vi "State_Queue_Driver.vi"(0 "Queue_Name_In":string, 1 "Max_Queue_Size_In":i32=-1, 5 "State_In":string, 7 "N_State_In":string[](array[string]), 9 "Time_Out_In_ms (10)":i32=10, 11 "Error_In":errorcluster, 13 "Queue_Operation":T1=enum."Flush") -> (3 "Max_Queue_Size_Out":i32=-1, 4 "Queue_Name_Out":string, 6 "State_Out":string, 15 "Error_Out":errorcluster)   [LabVIEW 2021]
doc: "Used to transfer data from one state to another."
uses:
  Controls/Queue_Driver_Select.ctl
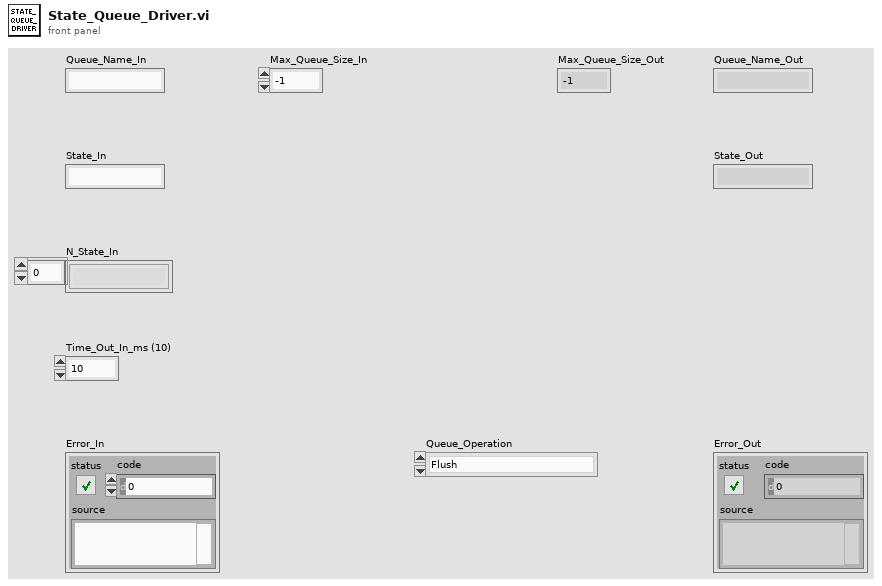
[diagram p1: front panel]
types:
  T1 = typedef "Queue_Driver_Select.ctl" = enum16{"Obtain_Queue", "Enqueue", "Enqueue_N", "Enqueue_at_Opposite_End", "Preview", "Queue_Status", "Dequeue", "Flush", "Release_Queue"}
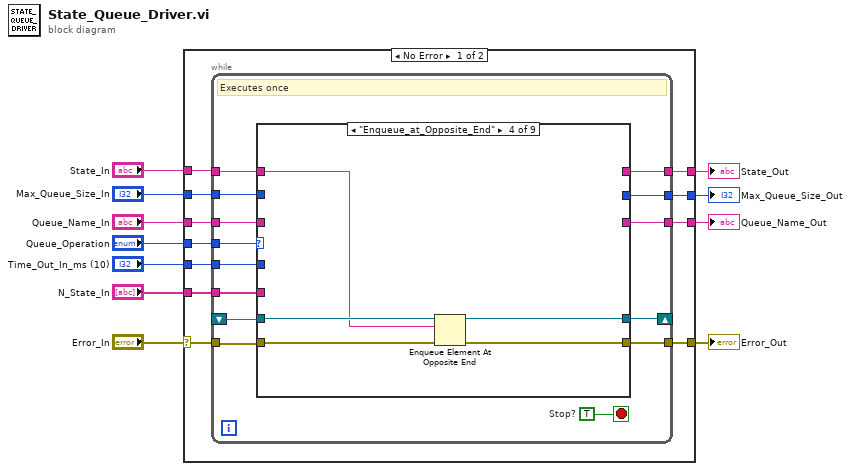
[diagram p0: block diagram]
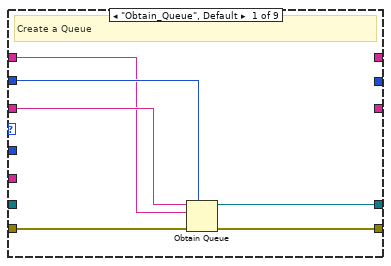
[diagram p2: hidden frame]
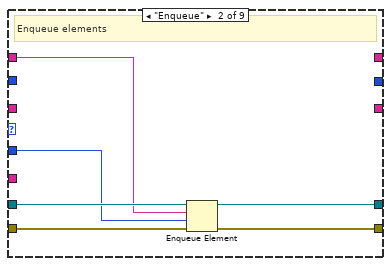
[diagram p3: hidden frame]
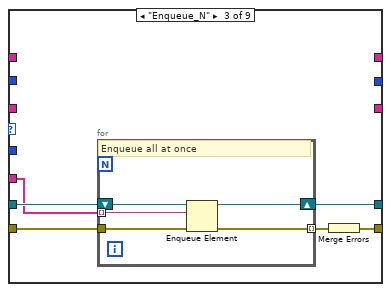
[diagram p4: hidden frame]
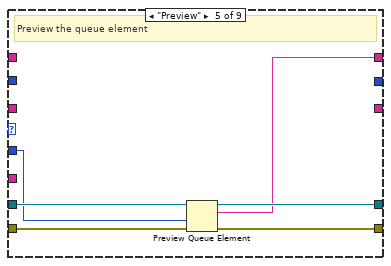
[diagram p5: hidden frame]
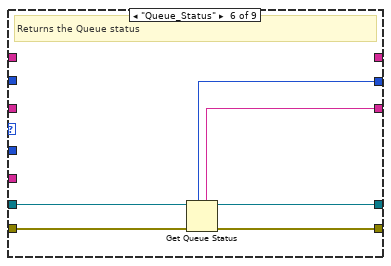
[diagram p6: hidden frame]
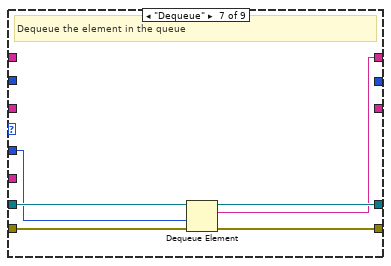
[diagram p7: hidden frame]
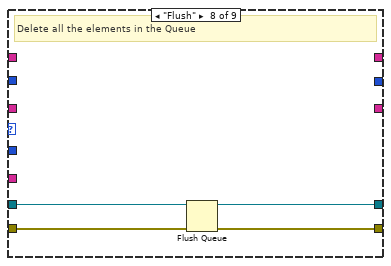
[diagram p8: hidden frame]
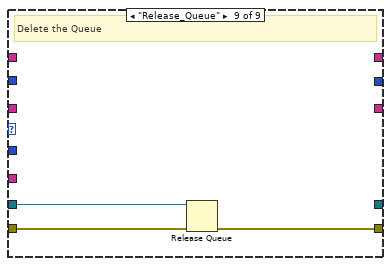
[diagram p9: hidden frame]
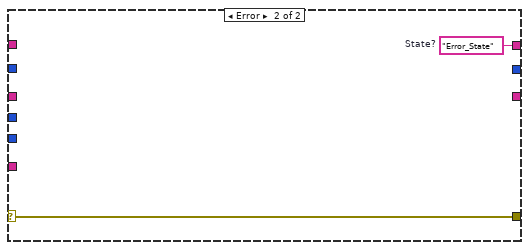
[diagram p10: hidden frame]
diagram:
  n1 = case shown="No Error" "Error_In" {
    selector: "Error_In" -> [w12 w91]
    tunnel: "Max_Queue_Size_In" -> [w22 _]
    tunnel: [w21 w91] -> w10
    tunnel: "Time_Out_In_ms (10)" -> [w20 _]
    tunnel: [w19 _] -> w8
    tunnel: [w18 _] -> w7
    tunnel: "Queue_Operation" -> [w17 _]
    tunnel: "Queue_Name_In" -> [w16 _]
    tunnel: "State_In" -> [w15 _]
    tunnel: [w14 w90] -> w3
    tunnel: "N_State_In" -> [w13 _]
    frame No Error {
      n2 = while {
        tunnel: w22 -> [w36]
        tunnel: w20 -> [w33]
        tunnel: [w31] -> w19
        tunnel: w17 -> [w28]
        shift-right: [w29] -> _
        shift-left: _ -> [w25]
        tunnel: w12 -> [w26]
        tunnel: [w35] -> w21
        tunnel: w13 -> [w23]
        tunnel: w15 -> [w34]
        tunnel: [w32] -> w14
        tunnel: w16 -> [w27]
        tunnel: [w30] -> w18
        stop <- w24 stop-if-true
        w24 = TRUE  # Stop?
        # "Executes once"
        n3 = case shown="\"Enqueue_at_Opposite_End\"" w28 {
          tunnel: w26 -> [w42 w48 w50 w63 w69 w75 w81 w85 w88]
          tunnel: w27 -> [w40 _ _ _ _ _ _ _ _]
          tunnel: w36 -> [w39 _ _ _ _ _ _ _ _]
          tunnel: [w37 w44 w53 w62 w68 w74 w80 w84 _] -> w29
          tunnel: [w41 w47 w49 w61 w67 w73 w78 w83 w87] -> w35
          tunnel: w25 -> [_ w46 w54 w64 w70 w76 w82 w86 w89]
          tunnel: w34 -> [w38 w45 _ w60 _ _ _ _ _]
          tunnel: w33 -> [_ w43 _ _ w66 _ w77 _ _]
          tunnel: [_ _ _ _ w65 _ w79 _ _] -> w32
          tunnel: [_ _ _ _ _ w72 _ _ _] -> w31
          tunnel: [_ _ _ _ _ w71 _ _ _] -> w30
          tunnel: w23 -> [_ _ w51 _ _ _ _ _ _]
          frame "Obtain_Queue", Default {
            # "Create a Queue"
            n4 = Obtain Queue(max queue size (-1, unlimited)=w39, name (unnamed)=w40, element data type=w38, error in (no error)=w42) -> (queue out=w37:refnum<queue>, error out=w41:errorcluster)  [unwired: 1 in, 1 out]
          }
          frame "Enqueue" {
            # "Enqueue elements"
            n5 = Enqueue Element(queue=w46, element=w45, timeout in ms (-1)=w43, error in (no error)=w48) -> (queue out=w44:refnum<queue>, error out=w47:errorcluster)  [unwired: 1 out]
          }
          frame "Enqueue_N" {
            n6 = for {
              tunnel: w51 -> [w55] mode=indexing
              shift-right: [w57] -> w53
              shift-left: w54 -> [w59]
              tunnel: w50 -> [w58]
              tunnel: [w56] -> w52 mode=indexing
              # "Enqueue all at once"
              n7 = Enqueue Element(queue=w59, element=w55, error in (no error)=w58) -> (queue out=w57:refnum<queue>, error out=w56:errorcluster)  [unwired: 1 in, 1 out]
            }
            n8 = Merge Errors(w52) -> (w49:errorcluster)
          }
          frame "Enqueue_at_Opposite_End" {
            n9 = Enqueue Element At Opposite End(queue=w64, element=w60, error in (no error)=w63) -> (queue out=w62:refnum<queue>, error out=w61:errorcluster)  [unwired: 1 in, 1 out]
          }
          frame "Preview" {
            # "Preview the queue element"
            n10 = Preview Queue Element(queue=w70, timeout in ms (-1)=w66, error in (no error)=w69) -> (queue out=w68:refnum<queue>, element=w65:string, error out=w67:errorcluster)  [unwired: 1 out]
          }
          frame "Queue_Status" {
            # "Returns the Queue status"
            n11 = Get Queue Status(queue=w76, error in (no error)=w75) -> (queue out=w74:refnum<queue>, queue name=w71:string, max queue size=w72:i32, error out=w73:errorcluster)  [unwired: 1 in, 4 out]
          }
          frame "Dequeue" {
            # "Dequeue the element in the queue"
            n12 = Dequeue Element(queue=w82, timeout in ms (-1)=w77, error in (no error)=w81) -> (queue out=w80:refnum<queue>, element=w79:string, error out=w78:errorcluster)  [unwired: 1 out]
          }
          frame "Flush" {
            # "Delete all the elements in the Queue"
            n13 = Flush Queue(queue=w86, error in (no error)=w85) -> (queue out=w84:refnum<queue>, error out=w83:errorcluster)  [unwired: 1 out]
          }
          frame "Release_Queue" {
            # "Delete the Queue"
            n14 = Release Queue(queue=w89, error in (no error)=w88) -> (error out=w87:errorcluster)  [unwired: 1 in, 2 out]
          }
        }
      }
    }
    frame Error {
      w90 = "Error_State"  # State?
    }
  }
  "Error_Out" <- w10
  "Max_Queue_Size_Out" <- w8
  "Queue_Name_Out" <- w7
  "State_Out" <- w3
